vi "ATF-Pump-Create AO Waveform.vi"(7 "dt(sec)":dbl=2000.0, 9 "Size":i32, 10 "AO Channel Names":string[](array[string]), 11 "AO Values In":dbl[](array[numeric])) -> (3 "AO Waveform":waveform(dbl)[](array[waveform]))   [LabVIEW 2022 SP3]
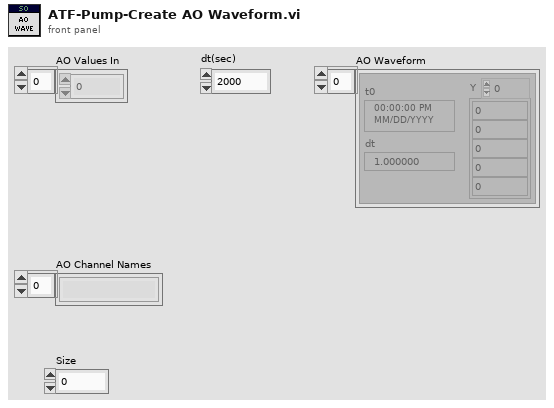
[diagram p1: front panel]
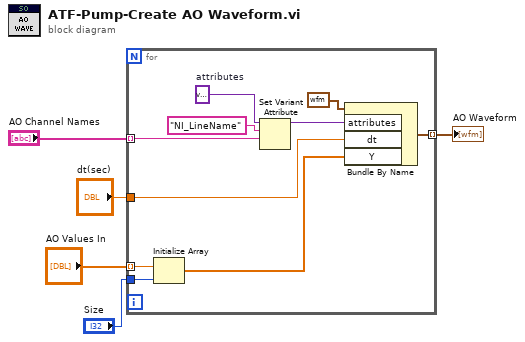
[diagram p0: block diagram]
diagram:
  n1 = for {
    tunnel: [w15] -> w3 mode=indexing
    tunnel: "Size" -> [w14]
    tunnel: "AO Values In" -> [w7] mode=indexing
    tunnel: "AO Channel Names" -> [w12] mode=indexing
    tunnel: "dt(sec)" -> [w9]
    w13 = variant  # attributes
    n2 = Initialize Array(w7, w14) -> (w6:dbl[])
    n3 = Set Variant Attribute(Variant=w13, name="NI_LineName", value=w12) -> (Variant out=w8:variant)  [unwired: 1 in, 2 out]
    n4 = Bundle By Name(cluster=waveform(dbl) {"t0"=timestamp(0 s since 1904-01-01), "dt"=1.0, "Y"=[]} ("waveform"), "attributes"=w8, "dt"=w9, "Y"=w6) -> (w15:waveform(dbl))
  }
  "AO Waveform" <- w3
